vi "噪声发生器DEMO.vi"() -> ()   [LabVIEW 2013]
panel:
  out "运行VI路径":path
  in  "停止":bool
  in  "插件VI":i32(listbox)
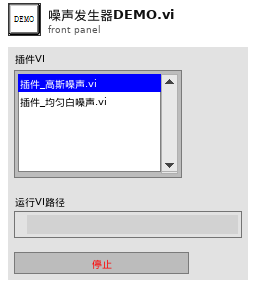
[diagram p1: front panel]
types:
  T1 = enum32{"Bad", "Idle", "Run top level", "Running"}
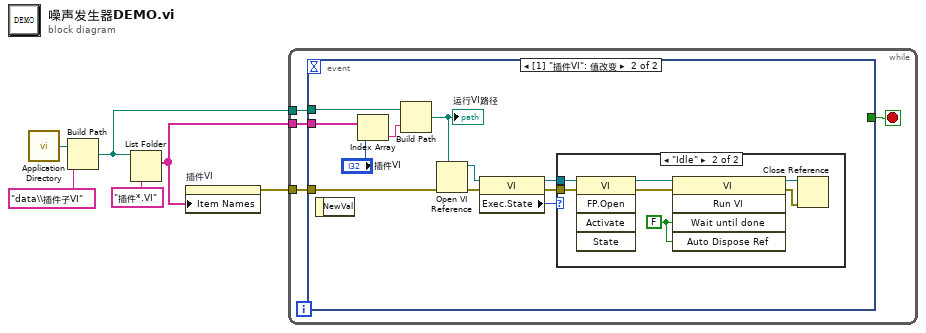
[diagram p0: block diagram]
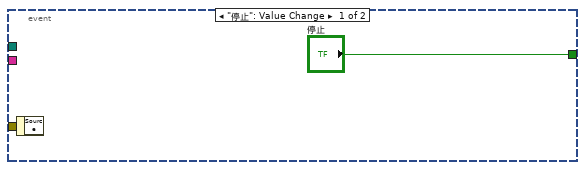
[diagram p2: hidden frame]
diagram:
  n1 = call <vilib>:"Application Directory.vi"() -> ("Application Directory"=w5:path)
  n2 = Build Path(base path=w5, name or relative path="data\\插件子VI" ("名称或相对路径")) -> (appended path=w3:path)
  n3 = List Folder(path=w3, pattern="插件*.VI" ("模式")) -> (filenames=w1:string[])  [unwired: 2 in, 3 out]
  n4 = property on="插件VI" class="LstBox (严格)"("Item Names"=w1) -> (error out=w6:errorcluster)  [unwired: 2 in, 1 out]
  n5 = while {
    tunnel: w6 -> [w8]
    tunnel: w3 -> [w9]
    tunnel: w1 -> [w7]
    stop <- w10 stop-if-true
    n6 = event shown="[1] \"插件VI\": 值改变" {
      selector: _ -> [_ _]
      dyn-events: _ -> [_ _]
      timeout: _ -> [_ _]
      tunnel: ["停止" _] -> w10
      tunnel: w9 -> [_ w21]
      tunnel: w8 -> [_ w15]
      tunnel: w7 -> [_ w13]
      event "停止": Value Change {
        n7 = event-data() -> ()  [unwired: 1 in, 1 out]
      }
      event "插件VI": Value Change {
        n8 = event-data() -> ()  [unwired: 1 in, 1 out]
        n9 = Index Array(array=w13, index="插件VI") -> (element=w12:string)
        n10 = Build Path(base path=w21, name or relative path=w12) -> (appended path=w20:path)
        "运行VI路径" <- w20
        n11 = Open VI Reference(vi path=w20, error in (no error)=w15) -> (vi reference=w18:refnum<vi>, error out=w19:errorcluster)  [unwired: 4 in]
        n12 = property class="VI"(reference=w18, error in=w19) -> (reference out=w16:refnum<vi>, error out=w14:errorcluster, "Exec.State"=w17:T1)
        n13 = case shown="\"Idle\"" w17 {
          tunnel: w16 -> [_ w29]
          tunnel: w14 -> [_ w28]
          frame "Bad", Default {
          }
          frame "Idle" {
            w23 = FALSE ("结束前等待")
            n14 = invoke class="VI" method="FP.Open"(reference=w29, error in=w28) -> (reference out=w27:refnum<vi>, error out=w26:errorcluster)  [unwired: 3 in, 3 out]
            n15 = invoke class="VI" method="Run VI"(reference=w27, error in=w26, "Wait until done"=w23, "Auto Dispose Ref"=w23) -> (reference out=w25:refnum<vi>, error out=w24:errorcluster)  [unwired: 1 in, 3 out]
            n16 = Close Reference(reference=w25, error in (no error)=w24) -> ()  [unwired: 1 out]
          }
        }
      }
    }
  }
